vi "AM PS Stop.vi"(11 "Queue in":refnum<queue>) -> ()   [LabVIEW 2020, in "Motion.lvlib"]
uses:
  Motion.lvlib
  support/Message Queue/Message Queue.lvlib
  support/Message Queue/Enqueue Message (Single).vi
  support/Message Queue/Message Cluster.ctl
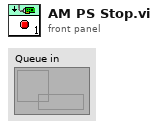
[diagram p1: front panel]
types:
  T1 = cluster{"Reset":bool, "PS Index":enum16{"PS 1", "PS 2", "PS 3", "PS 4"}}
  T2 = typedef "Message Queue.lvlib/Message Cluster.ctl" = cluster{"Message":string, "Message Data":variant}
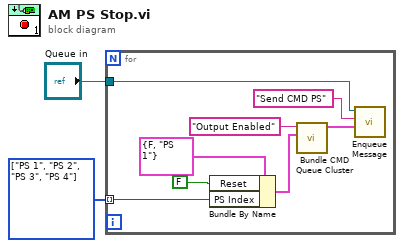
[diagram p0: block diagram]
diagram:
  w2 = enum16{"PS 1", "PS 2", "PS 3", "PS 4"}[] [enum."PS 1", enum."PS 2", enum."PS 3", enum."PS 4"] items=["PS 1", "PS 2", "PS 3", "PS 4"] ("PS Index")
  n1 = for {
    tunnel: "Queue in" -> [w10]
    tunnel: w2 -> [w3] mode=indexing
    n2 = Bundle By Name(cluster=T1 {"Reset"=FALSE, "PS Index"=enum."PS 1"} ("output cluster"), "Reset"=FALSE, "PS Index"=w3) -> (w5:T1)
    n3 = call "Bundle CMD Queue Cluster.vi"("Message Data"=w5, "Message"="Output Enabled") -> ("Message Cluster"=w7:T2)  [unwired: 9 in]
    n4 = call-poly "Enqueue Message.vi"("Message Data"=w7, "Message"="Send CMD PS", "Message Queue"=w10) -> ()  [unwired: 7 in, 2 out]
  }
